vi "测量数据解析-1001.vi"(11 "完整输入":string="\u0001\u0003\u0004\u0014\u0000\u0000\u0000ÿÃ") -> (0 "CRC？":bool, 2 "探头号":i32, 3 "测量值":dbl)   [LabVIEW 2017]
uses:
  <vilib>/regexp/Match Regular Expression.xnode
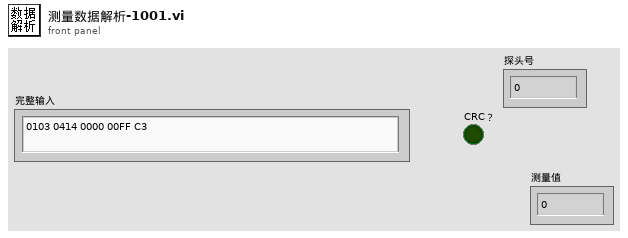
[diagram p1: front panel]
types:
  T1 = typedef "簇-输入.ctl" = cluster{"配置文件动作":T2, "数据输入":variant}
  T2 = typedef "枚举-配置文件动作.ctl" = enum16{"初始化加载配置", "读取配置", "写入-屏幕键盘", "写入-静音延迟", "写入-主要探头类型", "写入-串口配置", "写入-累积定时", "写入-导出定时", "保存配置到文件"}
  T3 = typedef "簇-配置文件内容.ctl" = cluster{"调试模式？":bool, "屏幕键盘？":bool, "软件版本":string, "静音延迟 s":u16, "主要探头类型":T4, "串口配置":cluster{"COM口":refnum<visa-resource-name>, "波特率":enum16{"9600", "19200"}, "读写超时ms":i16, "丢包判定次数":i16}, "定时配置-累积分段":T5, "定时配置-自动导出":cluster{"定时配置-自动导出":T5, "分别导出?":bool}}
  T4 = typedef "枚举-主要探头类型.ctl" = enum16{"网络探头", "串口探头"}
  T5 = typedef "簇-定时配置.ctl" = cluster{"定时模式":enum16{"绝对时间", "相对时间"}, "单位":enum16{"年", "月", "日", "时", "分"}, "间隔":u8, "目标时刻":timestamp}
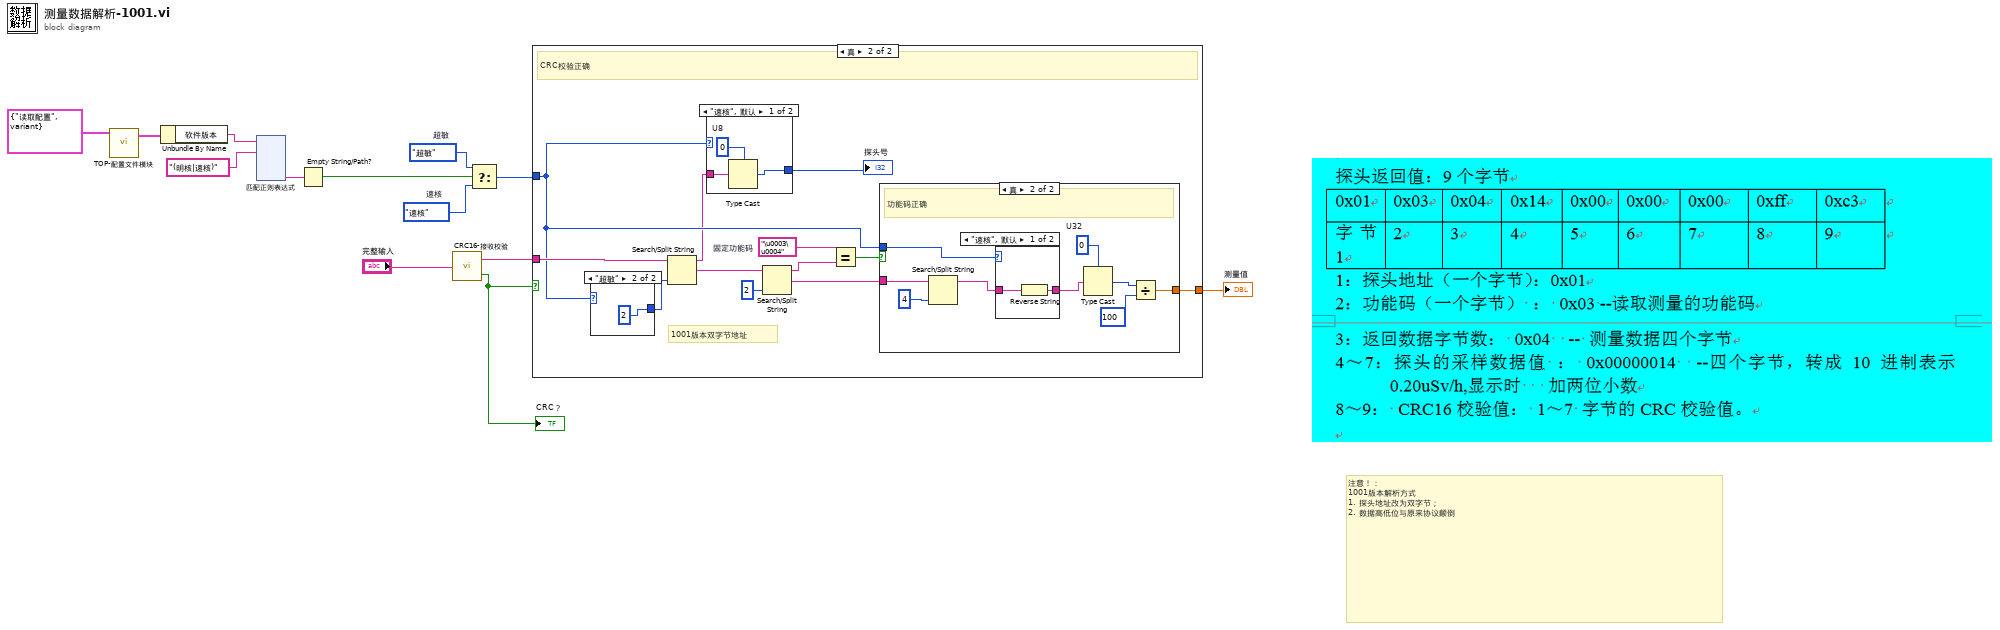
[diagram p0: block diagram]
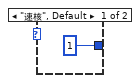
[diagram p3: hidden frame]
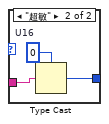
[diagram p4: hidden frame]
diagram:
  w9 = enum16{"速核", "超敏"}."速核"  # 速核
  w8 = enum16{"速核", "超敏"}."超敏"  # 超敏
  # "注意！：\n1001版本解析方式\n1. 探头地址改为双字节；\n2. 数据高低位与原来协议颠倒"
  n1 = call "TOP-配置文件模块.vi"("输入"=T1 {"配置文件动作"=enum."读取配置", "数据输入"=variant}) -> ("配置文件"=w4:T3)  [unwired: 9 in, 1 out]
  n2 = Unbundle By Name(w4) -> ("软件版本"=w3:string)
  n3 = xnode "匹配正则表达式"("输入字符串"=w3, "正则表达式"="(明核|速核)") -> ("子匹配 1"=w2:string)  [unwired: 4 in, 5 out]
  n4 = Empty String/Path?(string/path=w2) -> (empty?=w1:bool)
  n5 = call "CRC16-接收校验.vi"("读取缓冲区"="完整输入") -> ("净数据"=w12:string, "CRC？"=w11:bool)
  "CRC？" <- w11
  n6 = Select(t=w8, s=w1, f=w9) -> (s? t:f=w7:enum16{"速核", "超敏"})
  n7 = case shown="真" w11 {
    tunnel: w12 -> [_ w20]
    tunnel: [_ w23] -> w10
    tunnel: w7 -> [_ w16]
    frame False {
    }
    frame True {
      w21 = "\u0003\u0004"  # 固定功能码
      # "1001版本双字节地址"
      # "CRC校验正确"
      n8 = case shown="\"超敏\"" w16 {
        tunnel: [1 ("偏移量(0)") 2 ("偏移量(0)")] -> w17
        frame "速核", Default {
        }
        frame "超敏" {
        }
      }
      n9 = Search/Split String(string=w20, offset (0)=w17) -> (substring before match=w15:string, match + rest of string=w19:string)  [unwired: 1 in, 1 out]
      n10 = case shown="\"速核\", 默认" w16 {
        tunnel: w15 -> [w28 w33]
        tunnel: [w29 w31] -> w14
        frame "速核", Default {
          w30 = u8 0  # U8
          n11 = Type Cast(type=w30, x=w28) -> (*(type *) &x=w29:u8)
        }
        frame "超敏" {
          w32 = u16 0  # U16
          n12 = Type Cast(type=w32, x=w33) -> (*(type *) &x=w31:u16)
        }
      }
      "探头号" <- w14
      n13 = Search/Split String(string=w19, offset (0)=2 ("偏移量(0)")) -> (substring before match=w22:string, match + rest of string=w24:string)  [unwired: 1 in, 1 out]
      n14 = Equal?(x=w21, y=w22) -> (x = y?=w18:bool)
      n15 = case shown="真" w18 {
        tunnel: w24 -> [_ w42]
        tunnel: [_ w37] -> w23
        tunnel: w16 -> [_ w34]
        frame False {
        }
        frame True {
          w40 = u32 0  # U32
          # "功能码正确"
          n16 = Search/Split String(string=w42, offset (0)=4 ("偏移量(0)")) -> (substring before match=w36:string)  [unwired: 1 in, 2 out]
          n17 = case shown="\"速核\", 默认" w34 {
            tunnel: [w43 w45] -> w35
            tunnel: w36 -> [w44 w45]
            frame "速核", Default {
              n18 = Reverse String(1:w44) -> (0:w43:string)
            }
            frame "超敏" {
            }
          }
          n19 = Type Cast(type=w40, x=w35) -> (*(type *) &x=w39:u32)
          n20 = Divide(x=w39, y=u32 100) -> (x/y=w37:dbl)
        }
      }
    }
  }
  "测量值" <- w10
